vi "TestHighScores.vi"() -> ()   [LabVIEW 2020]
uses:
  TextDisplay Class.lvclass
  uiControlsMgr/uiControlsMgr.lvclass
panel:
  out "0009":string
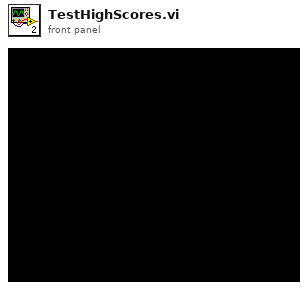
[diagram p1: front panel]
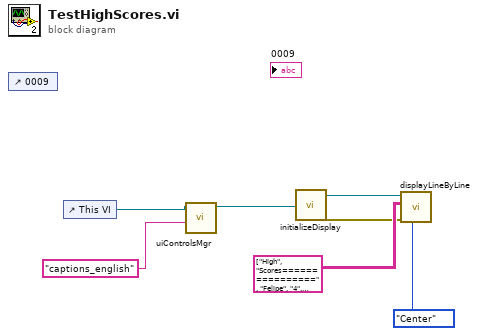
[diagram p0: block diagram]
diagram:
  n1 = control-ref of="0009"() -> ()  [unwired: 1 out]
  n2 = control-ref of="This VI"() -> (w2:refnum<vi>)
  n3 = call "uiControlsMgr.vi"("Captions File"="captions_english", "VI reference"=w2) -> ("uiControlsMgr out"=w3:refnum<class "uiControlsMgr.lvclass">)  [unwired: 8 in, 1 out]
  n4 = call "initializeDisplay.vi"("uiControlsMgr.lvclass"=w3) -> ("error out"=w5:errorcluster, "TextDisplay Class out"=w6:refnum<class "TextDisplay Class.lvclass">)  [unwired: 9 in]
  n5 = call "displayLineByLine.vi"("Justification"=enum16{"Left", "Center", "Right"}."Center", "error in (no error)"=w5, "scoreLog"=string[][] [["High", "Scores"], ["=========", "========="], ["Felipe", "4"], ["Lincoln", "6"], ["Plinio", "5"], ["Ligia", "9"], ["Belle", "4"]], "TextDisplay Class in"=w6) -> ()  [unwired: 6 in, 2 out]
